vi "Target Logging and Sampling Init.vi"(10 "error in (no error)":errorcluster) -> (2 "error out":errorcluster, 3 "Sampling Period (microsec)":i32=8333)   [LabVIEW 2018]
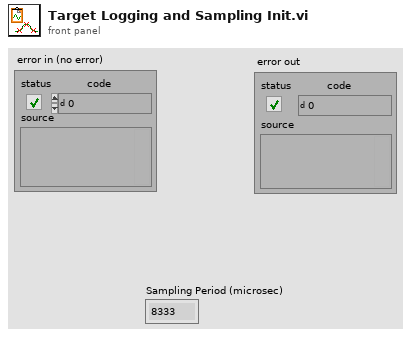
[diagram p1: front panel]
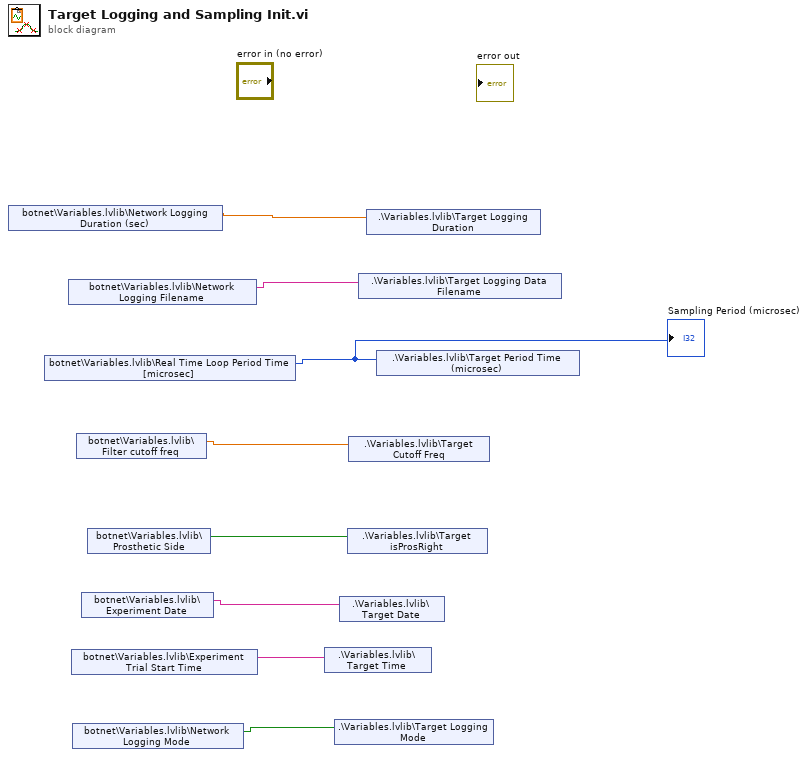
[diagram p0: block diagram]
diagram:
  n1 = shared-variable "botnet\\Variables.lvlib\\Network Logging Duration (sec)"() -> (w1:dbl)  [unwired: 1 in, 1 out]
  n2 = shared-variable "botnet\\Variables.lvlib\\Real Time Loop Period Time [microsec]"() -> (w8:u32)  [unwired: 1 in, 1 out]
  "Sampling Period (microsec)" <- w8
  n3 = shared-variable "botnet\\Variables.lvlib\\Network Logging Filename"() -> (w7:string)  [unwired: 1 in, 1 out]
  n4 = shared-variable "botnet\\Variables.lvlib\\Experiment Trial Start Time"() -> (w3:string)  [unwired: 1 in, 1 out]
  n5 = shared-variable "botnet\\Variables.lvlib\\Network Logging Mode"() -> (w2:bool)  [unwired: 1 in, 1 out]
  n6 = shared-variable "botnet\\Variables.lvlib\\Filter cutoff freq"() -> (w6:dbl)  [unwired: 1 in, 1 out]
  n7 = shared-variable "botnet\\Variables.lvlib\\Experiment Date"() -> (w4:string)  [unwired: 1 in, 1 out]
  n8 = shared-variable "botnet\\Variables.lvlib\\Prosthetic Side"() -> (w5:bool)  [unwired: 1 in, 1 out]
  n9 = shared-variable ".\\Variables.lvlib\\Target Time"(w3) -> ()  [unwired: 1 in, 1 out]
  n10 = shared-variable ".\\Variables.lvlib\\Target Logging Mode"(w2) -> ()  [unwired: 1 in, 1 out]
  n11 = shared-variable ".\\Variables.lvlib\\Target Date"(w4) -> ()  [unwired: 1 in, 1 out]
  n12 = shared-variable ".\\Variables.lvlib\\Target isProsRight"(w5) -> ()  [unwired: 1 in, 1 out]
  n13 = shared-variable ".\\Variables.lvlib\\Target Cutoff Freq"(w6) -> ()  [unwired: 1 in, 1 out]
  n14 = shared-variable ".\\Variables.lvlib\\Target Logging Data Filename"(w7) -> ()  [unwired: 1 in, 1 out]
  n15 = shared-variable ".\\Variables.lvlib\\Target Logging Duration"(w1) -> ()  [unwired: 1 in, 1 out]
  n16 = shared-variable ".\\Variables.lvlib\\Target Period Time (microsec)"(w8) -> ()  [unwired: 1 in, 1 out]
